vi "Untitled 2 (SubVI).vi"(4 "222":dbl, 5 "111":dbl, 6 "221":dbl, 7 "112":dbl, 8 "212":dbl, 9 "211":dbl, 10 "122":dbl, 11 "121":dbl) -> (3 "Array":dbl[][](array[numeric]))   [LabVIEW 2009]
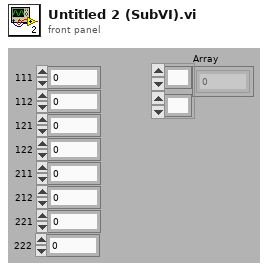
[diagram p1: front panel]
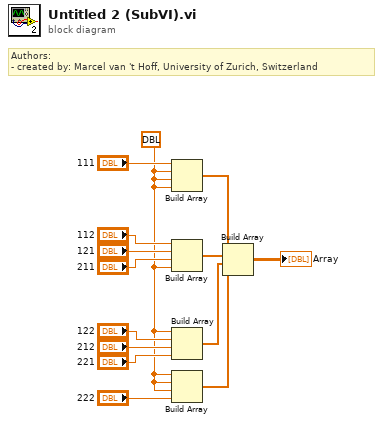
[diagram p0: block diagram]
diagram:
  w3 = dbl ? ("element")
  # "Authors: \n- created by: Marcel van 't Hoff, University of Zurich, Switzerland"
  n1 = Build Array("111", w3, w3, w3) -> (w13:dbl[])
  n2 = Build Array("112", "121", "211", w3) -> (w11:dbl[])
  n3 = Build Array(w3, "122", "212", "221") -> (w4:dbl[])
  n4 = Build Array(w3, w3, w3, "222") -> (w1:dbl[])
  n5 = Build Array(w13, w11, w4, w1) -> (→"Array":dbl[][])
